vi "Read Stored Sessions.vi"(11 "ConnectionHandler in":refnum<class "ConnectionHandler.lvclass">) -> (2 "Stored Sessions":refnum<class "Session.lvclass">[](array[class]), 3 "ConnectionHandler":refnum<class "ConnectionHandler.lvclass">)   [LabVIEW 2013, in "MQTT Server.lvlib" / "ConnectionHandler.lvclass"]
uses:
  ConnectionHandler.lvclass
  <vilib>/LabVIEW Open Source Project/MQTT Connection/MQTT_Base/Session/Session.lvclass
  ConnectionHandler.lvclass/ConnectionHandler.ctl
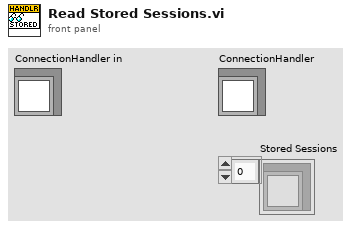
[diagram p1: front panel]
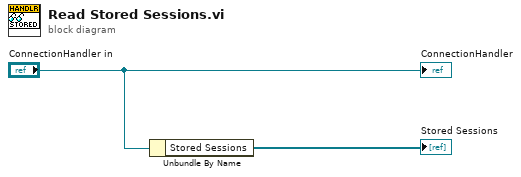
[diagram p0: block diagram]
diagram:
  n1 = Unbundle By Name("ConnectionHandler in") -> ("Stored Sessions"=→"Stored Sessions":refnum<class "Session.lvclass">[])
  "ConnectionHandler" <- "ConnectionHandler in"
